vi "build refresh token URI.vi"(8 "error in (no error)":errorcluster, 11 "Oauth2 in":refnum<class "Oauth2.lvclass">) -> (0 "error out":errorcluster, 2 "Refresh Token Request URI":string, 3 "Oauth2":refnum<class "Oauth2.lvclass">)   [LabVIEW 2013, in "Oauth2.lvclass"]
uses:
  Oauth2.lvclass
  OAuthToken/OAuth2 Token Element -- enum.ctl
  Oauth2.lvclass/Oauth2.ctl
  <vilib>/LabVIEW Open Source Project/OpenURI/uri/URI.lvclass
  OAuthToken/OAuthAccessToken.lvclass
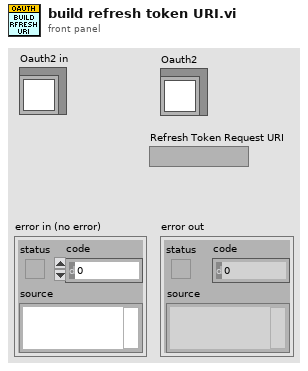
[diagram p1: front panel]
types:
  T1 = typedef "OAuthAccessToken.lvclass/OAuth2 Token Element -- enum.ctl" = enum16{"client_id", "client_secret", "response_type", "scope", "redirect_uri", "error", "error_description", "error_uri", "grant_type", "code", "access_token", "token_type", "expires_in", "username", "password", "refresh_token", "code_challenge", "code_verifier", "code_challenge_method", "endpoint element"}
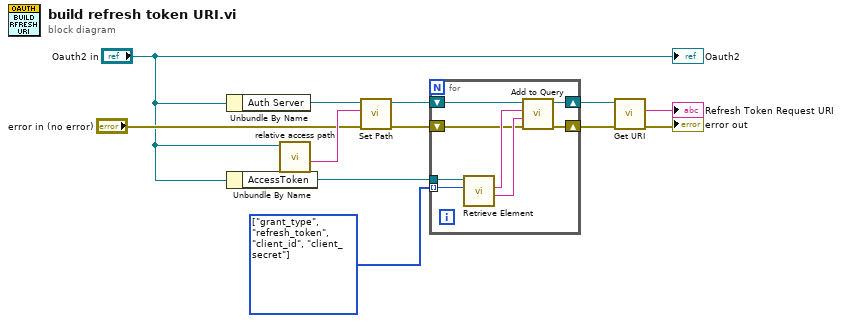
[diagram p0: block diagram]
diagram:
  w6 = T1[] [enum."grant_type", enum."refresh_token", enum."client_id", enum."client_secret"] items=["client_id", "client_secret", "response_type", "scope", "redirect_uri", "error", "error_description", "error_uri", "grant_type", "code", "access_token", "token_type", "expires_in", "username", "password", "refresh_token", "code_challenge", "code_verifier", "code_challenge_method", "endpoint element"]
  n1 = Unbundle By Name("Oauth2 in") -> ("Auth Server"=w9:refnum<class "URI.lvclass">)
  n2 = Unbundle By Name("Oauth2 in") -> ("AccessToken"=w7:refnum<class "OAuthAccessToken.lvclass">)
  n3 = call-dynamic "relative access path.vi"("Oauth2 in"="Oauth2 in") -> ("Token Access Path"=w10:string)  [unwired: 9 in, 1 out]
  n4 = call <vilib>:"Set Path.vi"("error in (no error)"="error in (no error)", "path"=w10, "URI in"=w9) -> ("error out"=w1:errorcluster, "URI out"=w4:refnum<class "URI.lvclass">)  [unwired: 7 in]
  n5 = for {
    tunnel: w7 -> [w20]
    tunnel: w6 -> [w19] mode=indexing
    shift-right: [w17] -> w3
    shift-left: w4 -> [w18]
    shift-right: [w13] -> w2
    shift-left: w1 -> [w14]
    n6 = call "Retrieve Element.vi"("Token element"=w19, "OAuthAccessToken in"=w20) -> ("Value"=w15:string, "Key"=w16:string)  [unwired: 6 in, 2 out]
    n7 = call <vilib>:"Add to Query.vi"("error in (no error)"=w14, "value"=w15, "key"=w16, "URI in"=w18) -> ("error out"=w13:errorcluster, "URI out"=w17:refnum<class "URI.lvclass">)  [unwired: 6 in]
  }
  n8 = call <vilib>:"Get URI.vi"("error in (no error)"=w2, "URI in"=w3) -> ("error out"=→"error out":errorcluster, "URI String"=→"Refresh Token Request URI":string)  [unwired: 7 in, 1 out]
  "Oauth2" <- "Oauth2 in"
